vi "PH_SHS_Analysis_Statistician.select Data.vi"(6 "Data Selector":i16, 8 "SHS Analyzer Dataset":T1 {"State" items=["no info", "off/false/out", "on/true/in", "Failure", "Alarm", "Status 1", "Status 2", "Status 3"]; "Zernicke Coefficients"."2nd Spherical" scale=-2.0..2.0 scale format="%.2f"; "Zernicke Coefficients"."2nd Coma y" scale=-2.0..2.0 scale format="%.2f"; "Zernicke Coefficients"."2nd Coma x" scale=-2.0..2.0 scale format="%.2f"; "Zernicke Coefficients"."2nd Astig 45°" scale=-2.0..2.0 scale format="%.2f"; "Zernicke Coefficients"."2nd Astig 0°" scale=-2.0..2.0 scale format="%.2f"; "Zernicke Coefficients"."Trefoil 30°" scale=-2.0..2.0 scale format="%.2f"; "Zernicke Coefficients"."Trefoil 0°" scale=-2.0..2.0 scale format="%.2f"; "Zernicke Coefficients"."Spherical" scale=-2.0..2.0 scale format="%.2f"; "Zernicke Coefficients"."Coma y" scale=-2.0..2.0 scale format="%.2f"; "Zernicke Coefficients"."Coma x" scale=-2.0..2.0 scale format="%.2f"; "Zernicke Coefficients"."Astig 45°" scale=-2.0..2.0 scale format="%.2f"; "Zernicke Coefficients"."Astig 0°" scale=-2.0..2.0 scale format="%.2f"; "Zernicke Coefficients"."Defocus" scale=-2.0..2.0 scale format="%.2f"; "Zernicke Coefficients"."Tilt y" scale=-2.0..2.0 scale format="%.2f"; "Zernicke Coefficients"."Tilt x" scale=-2.0..2.0 scale format="%.2f"}) -> (1 "Data chosen?":bool, 2 "Data Legend":string, 3 "Data":dbl)   [LabVIEW 2014, in "PH_SHS_Analysis_Statistician.lvlib"]
doc: "This VI selects the data to be indicated."
uses:
  PH_SHS_Analysis_Statistician.lvlib
  PH_SHS_Analysis/PH_SHS_Analysis.Zernike Dataset.ctl
  PH_Basics/PH_StatusHandler/PH_StatusHandler.Status.ctl
  PH_SHS_Analysis/PH_SHS_Analysis.Zernike Coefficients.ctl
  PH_SHS_Analysis/PH_SHS_Analysis.lvlib
  PH_Basics/PH_StatusHandler/PH_StatusHandler.lvlib
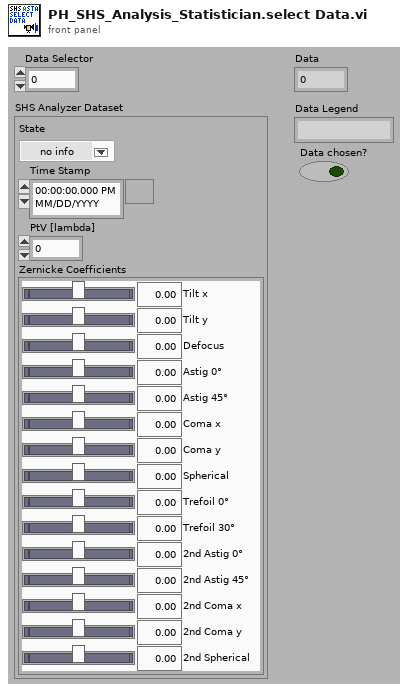
[diagram p1: front panel]
types:
  T1 = typedef "PH_SHS_Analysis.lvlib/PH_SHS_Analysis.Zernike Dataset.ctl" = cluster{"State":T2, "Time Stamp":timestamp, "PtV [lambda]":dbl, "Zernicke Coefficients":T3}
  T2 = typedef "PH_StatusHandler.lvlib/PH_StatusHandler.Status.ctl" = i16
  T3 = typedef "PH_SHS_Analysis.lvlib/PH_SHS_Analysis.Zernike Coefficients.ctl" = cluster{"Tilt x":dbl, "Tilt y":dbl, "Defocus":dbl, "Astig 0°":dbl, "Astig 45°":dbl, "Coma x":dbl, "Coma y":dbl, "Spherical":dbl, "Trefoil 0°":dbl, "Trefoil 30°":dbl, "2nd Astig 0°":dbl, "2nd Astig 45°":dbl, "2nd Coma x":dbl, "2nd Coma y":dbl, "2nd Spherical":dbl}
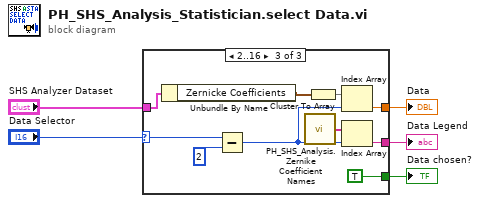
[diagram p0: block diagram]
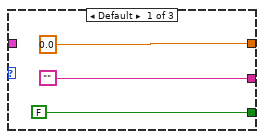
[diagram p2: hidden frame]
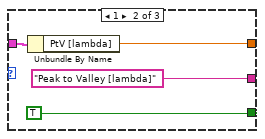
[diagram p3: hidden frame]
diagram:
  n1 = case shown="2..16" "Data Selector" {
    selector: "Data Selector" -> [_ _ w17]
    tunnel: [0.0 ("Maj FWHM") w12 w19] -> w5
    tunnel: ["" "Peak to Valley [lambda]" ("string") w14] -> w3
    tunnel: "SHS Analyzer Dataset" -> [_ w11 w22]
    tunnel: [FALSE TRUE TRUE] -> w2
    frame Default {
    }
    frame 1 {
      n2 = Unbundle By Name(w11) -> ("PtV [lambda]"=w12:dbl)
    }
    frame 2..16 {
      n3 = Unbundle By Name(w22) -> ("Zernicke Coefficients"=w21:T3)
      n4 = Subtract(x=w17, y=i16 2) -> (x-y=w15:i16)
      n5 = call "PH_SHS_Analysis.Zernike Coefficient Names.vi"() -> ("Zernickes"=w18:string[])
      n6 = Cluster To Array(cluster=w21) -> (array=w20:dbl[])
      n7 = Index Array(array=w20, index=w15) -> (element=w19:dbl)
      n8 = Index Array(array=w18, index=w15) -> (element=w14:string)
    }
  }
  "Data Legend" <- w3
  "Data chosen?" <- w2
  "Data" <- w5
